vi "Read Playbook Reference.vi"(8 "error in (no error)":errorcluster, 11 "Game in":refnum<class "Game.lvclass">) -> (0 "error out":errorcluster, 2 "Playbook Reference":refnum<data-value>, 3 "Game out":refnum<class "Game.lvclass">)   [LabVIEW 2022 SP3, in "Game.lvclass"]
uses:
  Game.lvclass
  Playbook_class/Playbook.lvclass
  Game.lvclass/Game.ctl
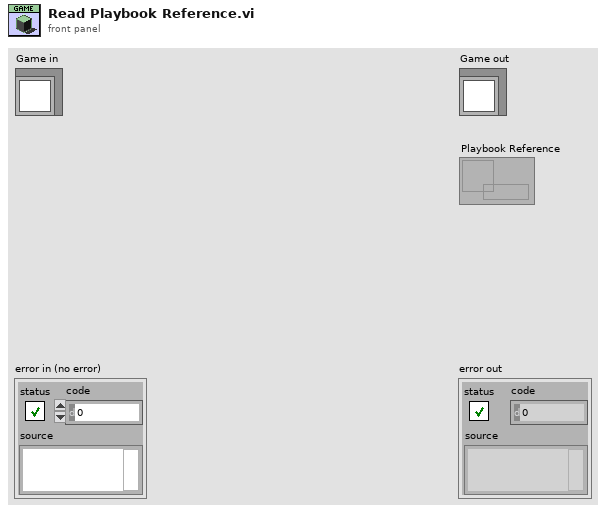
[diagram p1: front panel]
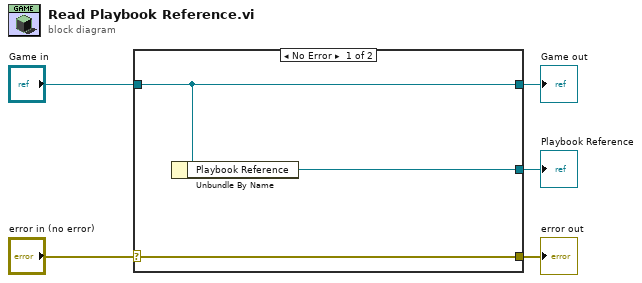
[diagram p0: block diagram]
diagram:
  n1 = case shown="No Error" "error in (no error)" {
    selector: "error in (no error)" -> [w8 w9]
    tunnel: [w8 w9] -> w4
    tunnel: [w7 w10] -> w2
    tunnel: "Game in" -> [w7 w10]
    tunnel: [w6 _] -> w1
    frame No Error {
      n2 = Unbundle By Name(w7) -> ("Playbook Reference"=w6:refnum<data-value>)
    }
    frame Error {
    }
  }
  "error out" <- w4
  "Game out" <- w2
  "Playbook Reference" <- w1
